vi "DisplayCurrentConfiguration.vi"(9 "error code  in":i32, 11 "Handle Cluster":T2) -> ()   [LabVIEW 2013, in "Gage.lvlib"]
uses:
  <instrlib>/GageLv_uic/Gage.lvlib
panel:
  in  "Triggers":u32
  in  "Channels":u32
  out "Channel":T1={"Coupling"="", "Differential Input"=FALSE, "Direct-to-ADC"=FALSE, "Impedance"=1000000, "Range"=1000, "DC Offset"=0, "Filter"=0} {"Impedance" min=50 max=1000000 step=999950 format="%.0p"}
  in  "Close":bool
  out "Trigger":T3={"Slope"="", "Level"=0, "Source"=0, "External Range"=10000, "External Coupling"="", "External Trigger"=FALSE, "Disable Trigger"=FALSE, "External Impedance"=""} {"External Range" min=2000 max=10000 step=8000; "Level" min=-100 max=100}
  out "Acquisition":T4={"Sample Rate"=100000000.0, "Mode"="", "Depth"=4096.0, "Segment Size"=4096.0, "Trigger Timeout"=1000.0, "Trigger Holdoff"=0.0, "Trigger Delay"=0.0, "Clock mode"=enum."Internal"} {"Sample Rate" format="%.0p"}
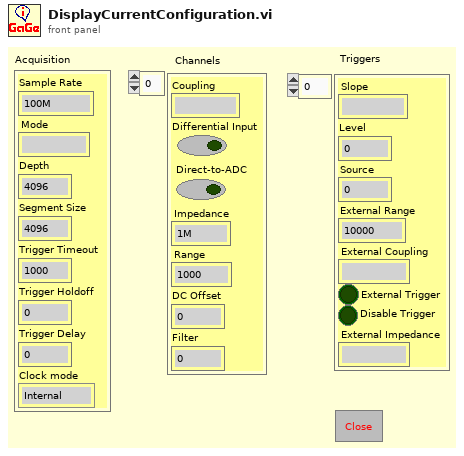
[diagram p1: front panel]
types:
  T1 = cluster{"Coupling":string, "Differential Input":bool, "Direct-to-ADC":bool, "Impedance":u32, "Range":u32, "DC Offset":i32, "Filter":u32}
  T2 = cluster{"Handle":u32, "Bits":u32, "Resolution":i32, "Offset":i32, "Channels":u32, "Boards":u32}
  T3 = cluster{"Slope":string, "Level":i32, "Source":i32, "External Range":u32, "External Coupling":string, "External Trigger":bool, "Disable Trigger":bool, "External Impedance":string}
  T4 = cluster{"Sample Rate":dbl, "Mode":string, "Depth":dbl, "Segment Size":dbl, "Trigger Timeout":dbl, "Trigger Holdoff":dbl, "Trigger Delay":dbl, "Clock mode":enum16{"Internal", "External", "Reference"}}
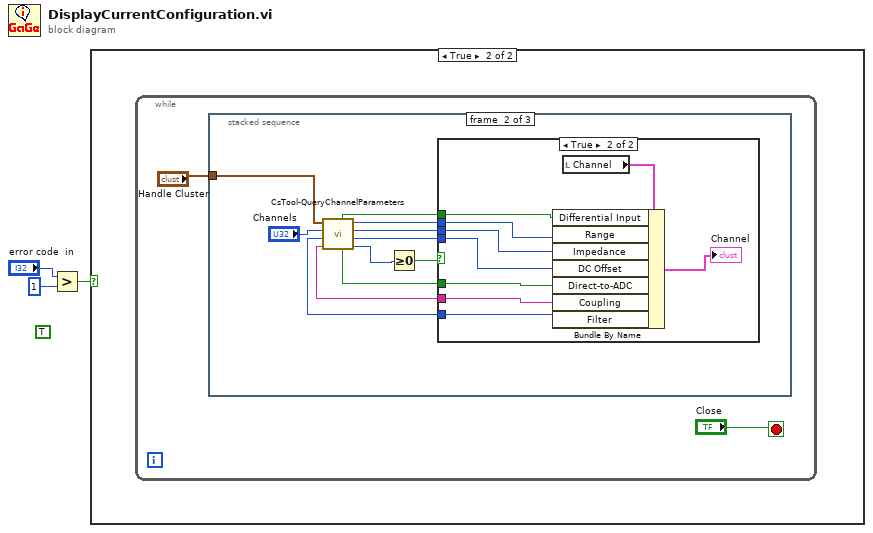
[diagram p0: block diagram]
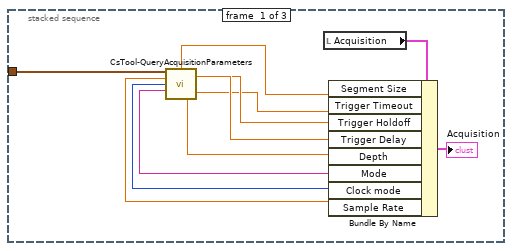
[diagram p3: hidden frame]
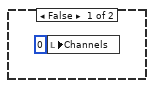
[diagram p4: hidden frame]
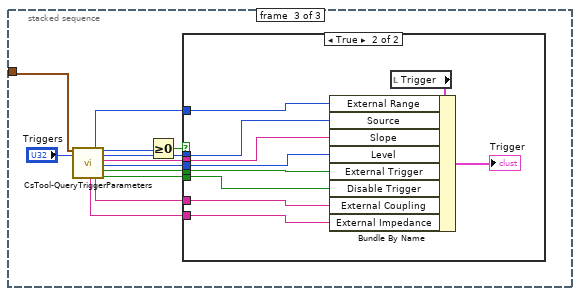
[diagram p5: hidden frame]
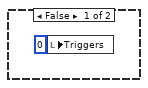
[diagram p6: hidden frame]
diagram:
  (unwired) TRUE
  n1 = Greater?(x="error code  in", y=1) -> (0:w1:bool)
  n2 = case shown="True" w1 {
    frame False {
    }
    frame True {
      n3 = while {
        stop <- "Close" stop-if-true
        n4 = stacked-sequence {
          tunnel: "Handle Cluster" -> [w6 w19 w46]
          frame #0 {
            n5 = call <instrlib>:"CsTool-QueryAcquisitionParameters.vi"("Handle Cluster"=w6) -> ("Trigger Holdoff"=w9:dbl, "Trigger Delay"=w10:dbl, "Sample Rate"=w14:dbl, "Clock Mode"=w13:enum16{"Internal", "External", "Reference"}, "Mode"=w12:string, "Trigger Timeout"=w8:dbl, "Segment Size"=w7:dbl, "Depth"=w11:dbl)  [unwired: 4 in, 3 out]
            n6 = local read "Acquisition"() -> (w16:T4)
            n7 = Bundle By Name(cluster=w16, "Segment Size"=w7, "Trigger Timeout"=w8, "Trigger Holdoff"=w9, "Trigger Delay"=w10, "Depth"=w11, "Mode"=w12, "Clock mode"=w13, "Sample Rate"=w14) -> (→"Acquisition":T4)
          }
          frame #1 {
            n8 = call <instrlib>:"CsTool-QueryChannelParameters.vi"("Handle Cluster"=w19, "Channel"="Channels") -> ("Filter"=w18:u32, "Coupling"=w23:string, "Differential Input"=w27:bool, "Direct-to-ADC"=w17:bool, "Range (mV)"=w26:u32, "Impedance"=w25:u32, "DC Offset (mV)"=w24:u32, "Error Code"=w21:i32)
            n9 = Greater Or Equal To 0?(x=w21) -> (x >= 0?=w20:bool)
            n10 = case shown="True" w20 {
              tunnel: w27 -> [_ w36]
              tunnel: w26 -> [_ w35]
              tunnel: w25 -> [_ w34]
              tunnel: w24 -> [_ w33]
              tunnel: w23 -> [_ w32]
              tunnel: w18 -> [_ w30]
              tunnel: w17 -> [_ w29]
              frame False {
                n11 = local write "Channels"(u32 0 ("Channels")) -> ()
              }
              frame True {
                n12 = local read "Channel"() -> (w31:T1)
                n13 = Bundle By Name(cluster=w31, "Differential Input"=w36, "Range"=w35, "Impedance"=w34, "DC Offset"=w33, "Direct-to-ADC"=w29, "Coupling"=w32, "Filter"=w30) -> (→"Channel":T1)
              }
            }
          }
          frame #2 {
            n14 = call <instrlib>:"CsTool-QueryTriggerParameters.vi"("Handle Cluster"=w46, "Trigger"="Triggers") -> ("External Impedance"=w38:string, "External Range (mV)"=w43:u32, "External Coupling"=w39:string, "Error Code"=w49:i32, "Source"=w42:i32, "Slope"=w41:string, "Level"=w40:i32, "External Trigger"=w44:bool, "Disable Trigger"=w45:bool)  [unwired: 9 in]
            n15 = Greater Or Equal To 0?(x=w49) -> (x >= 0?=w48:bool)
            n16 = case shown="True" w48 {
              tunnel: w45 -> [_ w53]
              tunnel: w44 -> [_ w54]
              tunnel: w43 -> [_ w58]
              tunnel: w42 -> [_ w57]
              tunnel: w41 -> [_ w56]
              tunnel: w40 -> [_ w55]
              tunnel: w39 -> [_ w52]
              tunnel: w38 -> [_ w51]
              frame False {
                n17 = local write "Triggers"(u32 0 ("Triggers")) -> ()
              }
              frame True {
                n18 = local read "Trigger"() -> (w59:T3)
                n19 = Bundle By Name(cluster=w59, "External Range"=w58, "Source"=w57, "Slope"=w56, "Level"=w55, "External Trigger"=w54, "Disable Trigger"=w53, "External Coupling"=w52, "External Impedance"=w51) -> (→"Trigger":T3)
              }
            }
          }
        }
      }
    }
  }
